vi "GenerateScanEndPtsLengthRound.vi"(0 "X Start":sgl, 1 "Mode":enum16{"Raster", "Serpentine"}(ring), 2 "Calibration":cluster{dbl, "MicrostepMode":u32}[](array[cluster]), 5 "X End":sgl=9.0, 7 "Y Start":sgl, 9 "Y End":sgl=10.0, 11 "error in":errorcluster, 12 "Y Step":sgl=6.0, 13 "X Step":sgl=6.0) -> (4 "Coordinate Array":sgl[][](array[numeric]), 6 "X Pixel Count":u64, 8 "Step Sizes":sgl[](array[numeric]), 10 "Y Pixel Count":u64, 15 "error out":errorcluster)   [LabVIEW 2020]
panel:
  out "Pixel Map":cluster{dbl[], dbl[]}(graph)
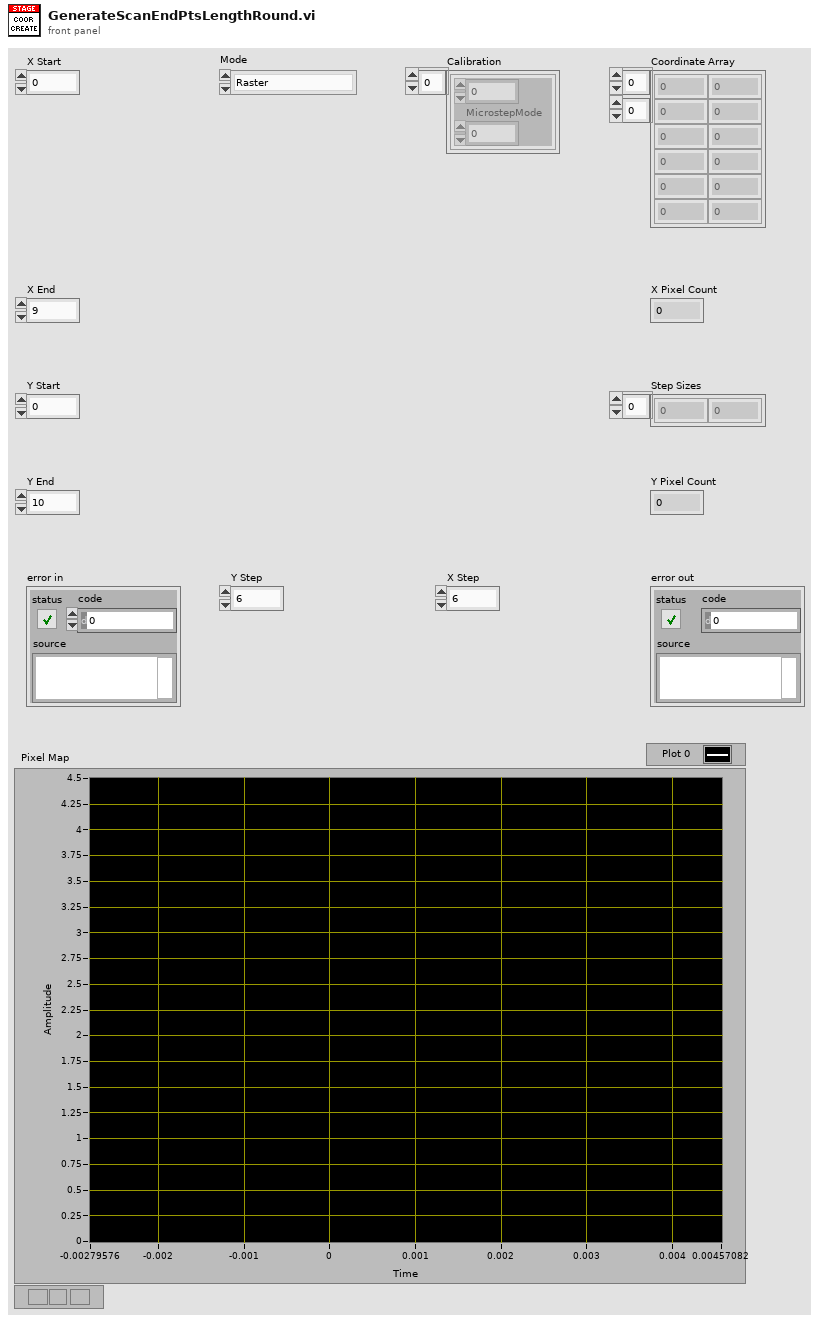
[diagram p1: front panel]
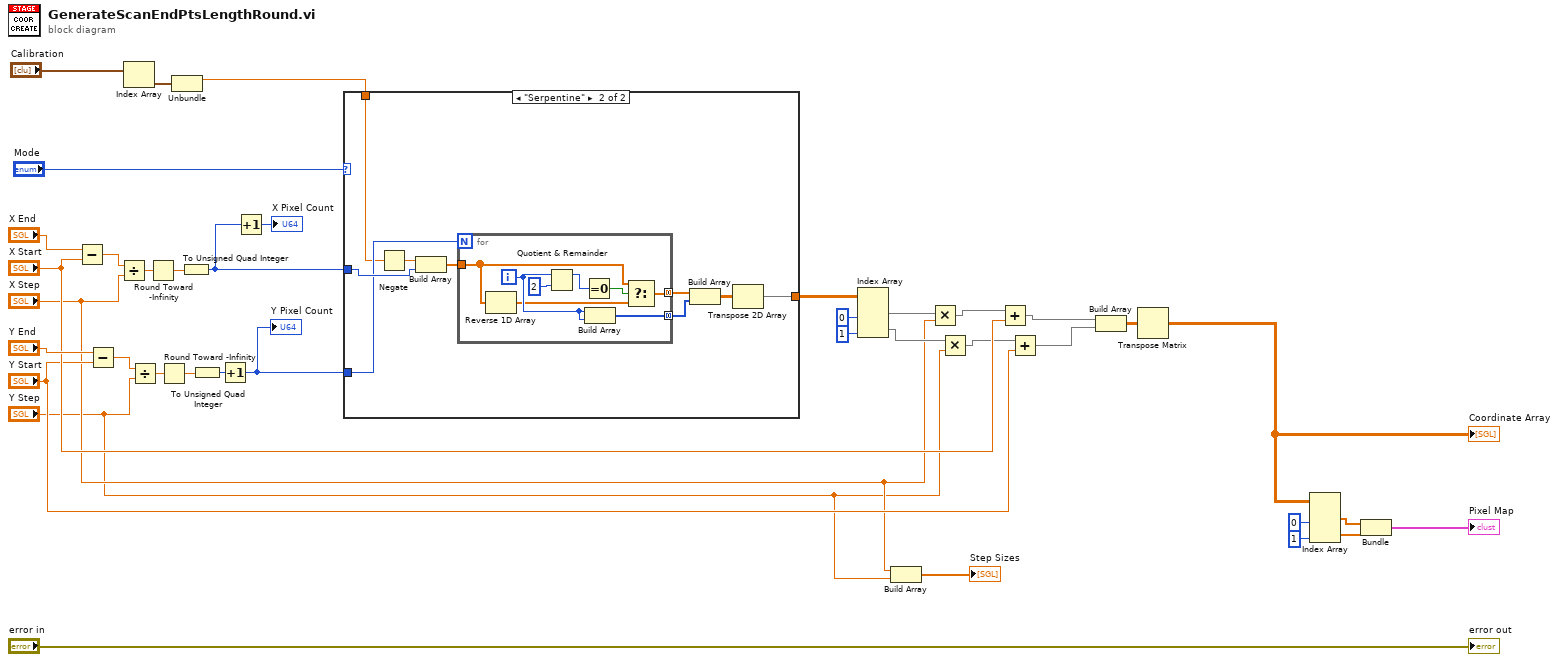
[diagram p0: block diagram]
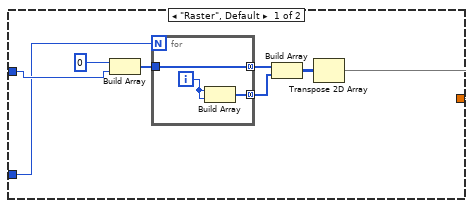
[diagram p2: hidden frame]
diagram:
  n1 = Subtract(x="X End", y="X Start") -> (x-y=w31:sgl)
  n2 = Subtract(x="Y End", y="Y Start") -> (x-y=w26:sgl)
  n3 = Divide(x=w31, y="X Step") -> (x/y=w30:sgl)
  n4 = Index Array(array="Calibration") -> (element=w2:cluster{dbl, "MicrostepMode":u32})  [unwired: 1 in]
  n5 = Divide(x=w26, y="Y Step") -> (x/y=w27:sgl)
  n6 = Round Toward -Infinity(1:w30) -> (0:w29:sgl)
  n7 = Round Toward -Infinity(1:w27) -> (0:w28:sgl)
  n8 = Unbundle(w2) -> (w1:dbl)  [unwired: 1 out]
  n9 = To Unsigned Quad Integer(1:w29) -> (0:w23:u64)
  n10 = To Unsigned Quad Integer(1:w28) -> (0:w24:u64)
  n11 = Increment(x=w24) -> (x+1=w5:u64)
  "Y Pixel Count" <- w5
  n12 = Increment(x=w23) -> (x+1=→"X Pixel Count":u64)
  n13 = case shown="\"Serpentine\"" "Mode" {
    tunnel: w23 -> [w45 w58]
    tunnel: w5 -> [w43 w56]
    tunnel: [w39 w52] -> w22
    tunnel: w1 -> [_ w51]
    frame "Raster", Default {
      n14 = Build Array(u64 0 ("element"), w45) -> (w44:u64[])
      n15 = for {
        N: w43 -> [_]
        tunnel: w44 -> [w49]
        tunnel: [w49] -> w41 mode=concatenating
        tunnel: [w47] -> w40 mode=concatenating
        i -> [w48]
        n16 = Build Array(w48, w48) -> (w47:i32[])
      }
      n17 = Build Array(w41, w40) -> (w42:u64[][])
      n18 = Transpose 2D Array(2D array=w42) -> (transposed array=w39:u64[][])
    }
    frame "Serpentine" {
      n19 = Negate(x=w51) -> (-x=w50:dbl)
      n20 = Build Array(w50, w58) -> (w57:dbl[])
      n21 = for {
        N: w56 -> [_]
        tunnel: w57 -> [w60]
        tunnel: [w65] -> w54 mode=concatenating
        tunnel: [w66] -> w53 mode=concatenating
        i -> [w64]
        n22 = Reverse 1D Array(array=w60) -> (reversed array=w59:dbl[])
        n23 = Quotient & Remainder(x=w64, y=2) -> (x-y*floor(x/y)=w62:i32)  [unwired: 1 out]
        n24 = Equal To 0?(x=w62) -> (x = 0?=w61:bool)
        n25 = Build Array(w64, w64) -> (w66:i32[])
        n26 = Select(t=w60, s=w61, f=w59) -> (s? t:f=w65:dbl[])
      }
      n27 = Build Array(w54, w53) -> (w55:dbl[][])
      n28 = Transpose 2D Array(2D array=w55) -> (transposed array=w52:dbl[][])
    }
  }
  n29 = Index Array(array=w22, index (col) #1=0 ("disabled index (col)"), index (col) #2=1 ("index (col)")) -> (element #1=w19:dbl[], element #2=w15:dbl[])  [unwired: 2 in]
  n30 = Build Array("X Step", "Y Step") -> (→"Step Sizes":sgl[])
  n31 = Multiply(x=w19, y="X Step") -> (x*y=w17:dbl[])
  n32 = Multiply(x=w15, y="Y Step") -> (x*y=w16:dbl[])
  n33 = Add(x=w17, y="X Start") -> (x+y=w13:dbl[])
  n34 = Add(x=w16, y="Y Start") -> (x+y=w12:dbl[])
  n35 = Build Array(w13, w12) -> (w11:dbl[][])
  n36 = Transpose Matrix(1:w11) -> (0:w4:dbl[][])
  "Coordinate Array" <- w4
  n37 = Index Array(array=w4, index (col) #1=0 ("disabled index (col)"), index (col) #2=1 ("index (col)")) -> (element #1=w36:dbl[], element #2=w35:dbl[])  [unwired: 2 in]
  n38 = Bundle(w36, w35) -> (→"Pixel Map":cluster{dbl[], dbl[]})  [unwired: 1 in]
  "error out" <- "error in"
